vi "Initiate Updates.vi"(8 "error in (no error)":errorcluster, 11 "IViewModel In":refnum<class "IViewModel.lvclass">) -> (0 "error out":errorcluster, 3 "IViewModel Out":refnum<class "IViewModel.lvclass">)   [LabVIEW 2015, in "IViewModel.lvlib" / "IViewModel.lvclass"]
doc: "<License>\nCopyright © 2017 Composed Systems, LLC | All rights reserved\nwww.composed.io\n\nAuthor: Ethan Stern <ethan.stern@composed.io>\n\nThis software is provided \"AS IS\" WITHOUT WARRANTIES, either express or implied, AND IS FOR EDUCATIONAL PURPOSES ONLY.\n</License>"
uses:
  IViewModel.lvclass
  IViewable/IViewable/IViewable.lvclass/IViewable.ctl
  IViewManager/IViewManager/IViewManager.lvclass
  IViewable/IViewable/IViewable.lvclass
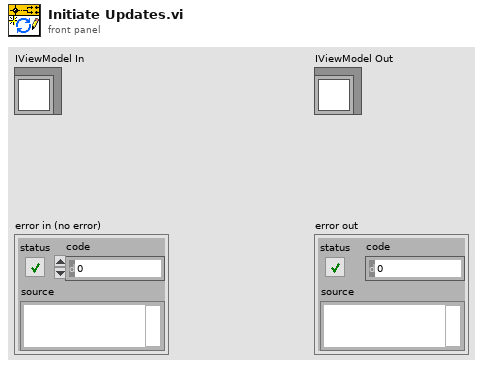
[diagram p1: front panel]
types:
  T1 = enum32{"Invalid", "Standard", "Closed", "Hidden", "Minimized", "Maximized"}
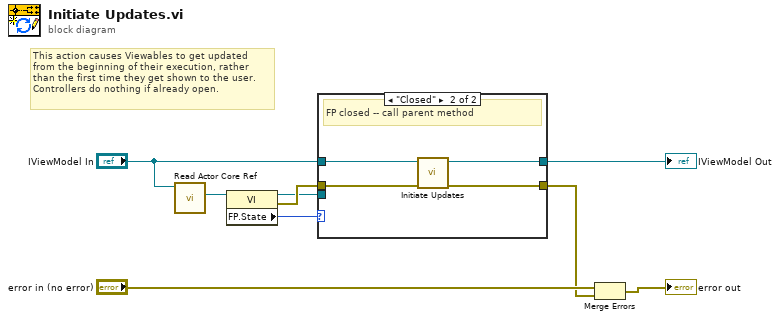
[diagram p0: block diagram]
diagram:
  # "This action causes Viewables to get updated\nfrom the beginning of their execution, rather\nthan the first time they get shown to the user.\nControllers do nothing if already open."
  n1 = call "Read Actor Core Ref.vi"("IViewable In"="IViewModel In") -> ("Actor Core Ref"=w7:refnum<vi>)  [unwired: 8 in, 2 out]
  n2 = property class="VI"(reference=w7) -> (reference out=w1:refnum<vi>, error out=w2:errorcluster, "FP.State"=w4:T1)  [unwired: 1 in]
  n3 = case shown="\"Closed\"" w4 {
    tunnel: "IViewModel In" -> [w11 w15]
    tunnel: [w11 w14] -> w5
    tunnel: [w10 w13] -> w3
    tunnel: w2 -> [w10 w12]
    tunnel: w1 -> [_ _]
    frame Default {
      # "FP not closed -- do nothing"
    }
    frame "Closed" {
      # "FP closed -- call parent method"
      n4 = call-parent "Initiate Updates.vi"("error in (no error)"=w12, "IViewable In"=w15) -> ("error out"=w13:errorcluster, "IViewable Out"=w14:refnum<class "IViewModel.lvclass">)  [unwired: 8 in]
    }
  }
  "IViewModel Out" <- w5
  n5 = Merge Errors("error in (no error)", w3) -> (→"error out":errorcluster)
